vi "Calc_GaussianNoise.vi"(8 "SD":dbl=1.0, 11 "Start Position":dbl) -> (3 "Final Position":dbl)   [LabVIEW 2020]
uses:
  <vilib>/gmath/statdist.llb/Normal Random.vi
  <vilib>/gmath/NI_Gmath.lvlib
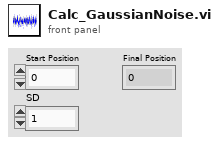
[diagram p1: front panel]
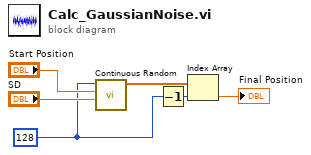
[diagram p0: block diagram]
diagram:
  w3 = 128 ("Trial")
  n1 = call-poly <vilib>:"Continuous Random.vi"("std"="SD", "mean"="Start Position", "samples"=w3) -> ("normal random data"=w4:dbl[])  [unwired: 7 in, 1 out]
  n2 = Decrement(x=w3) -> (x-1=w2:i32)
  n3 = Index Array(array=w4, index=w2) -> (element=→"Final Position":dbl)
